vi "read_data (SubVI).vi"(0 "VISA resource name":refnum<visa-resource-name>, 1 "Scope only?":bool=TRUE, 2 "Channels":i32[](array[ring]) items=["Channel 1"=0, "Channel 2"=1, "Channel 3"=2, "Channel 4"=3, "Waveform Memory 1"=5, "Waveform Memory 2"=6, "Serial Bus 1"=7, "Serial Bus 2"=8, "Digital Bus Low"=9, "Digital Bus High "=10, "Digital Bus 1"=11, "Digital Bus 2"=12, "Function 1"=32, "Function 2"=33, "Function 3"=34, "Function 4"=35, "Math 1"=36, "Math 2"=37, "Math 3"=38, "Math 4"=39], 5 "Use osciloscope chan 1":bool, 8 "index (row)":i32, 9 "error in (no error)":errorcluster, 11 "data tasks":T1) -> (4 "output data tasks":T3, 6 "Output data":dbl[][](array[numeric]), 7 "Output ASD 1":cluster{"f0":dbl, "df":dbl, "magnitude":dbl[]}[](array[cluster]), 10 "sample rate":dbl, 12 "Rescaled data":i16[][](array[numeric]), 13 "Output ASD 2":cluster{"f0":dbl, "df":dbl, "magnitude":dbl[]}, 14 "error out":errorcluster, 15 "VISA resource name out":refnum<visa-resource-name>)   [LabVIEW 2018]
uses:
  <vilib>/measure/maspectr.llb/Power Spectrum and PSD Export Mode.ctl
  <vilib>/DAQmx/read.llb/DAQmx Read (Analog 2D DBL NChan NSamp).vi
  <vilib>/DAQmx/miscellaneous.llb/DAQmx Fill In Error Info.vi
  <vilib>/measure/maspectr.llb/FFT Power Spectrum and PSD for 1 Chan.vi
  <vilib>/measure/NI_MAPro.lvlib
panel:
  in  "export mode 3":T2 items=["Power Spectrum", "Power Spectral Density"]
  in  "export mode 2":T2 items=["Power Spectrum", "Power Spectral Density"]
  in  "export mode":T2 items=["Power Spectrum", "Power Spectral Density"]
  out "error out 3":errorcluster
  out "VISA resource name out 3":refnum<visa-resource-name>
  in  "error in (no error) 3":errorcluster
  in  "Channels 3":i32[](array[ring]) items=["Channel 1"=0, "Channel 2"=1, "Channel 3"=2, "Channel 4"=3, "Waveform Memory 1"=5, "Waveform Memory 2"=6, "Serial Bus 1"=7, "Serial Bus 2"=8, "Digital Bus Low"=9, "Digital Bus High "=10, "Digital Bus 1"=11, "Digital Bus 2"=12, "Function 1"=32, "Function 2"=33, "Function 3"=34, "Function 4"=35, "Math 1"=36, "Math 2"=37, "Math 3"=38, "Math 4"=39]
  in  "VISA resource name 3":refnum<visa-resource-name>
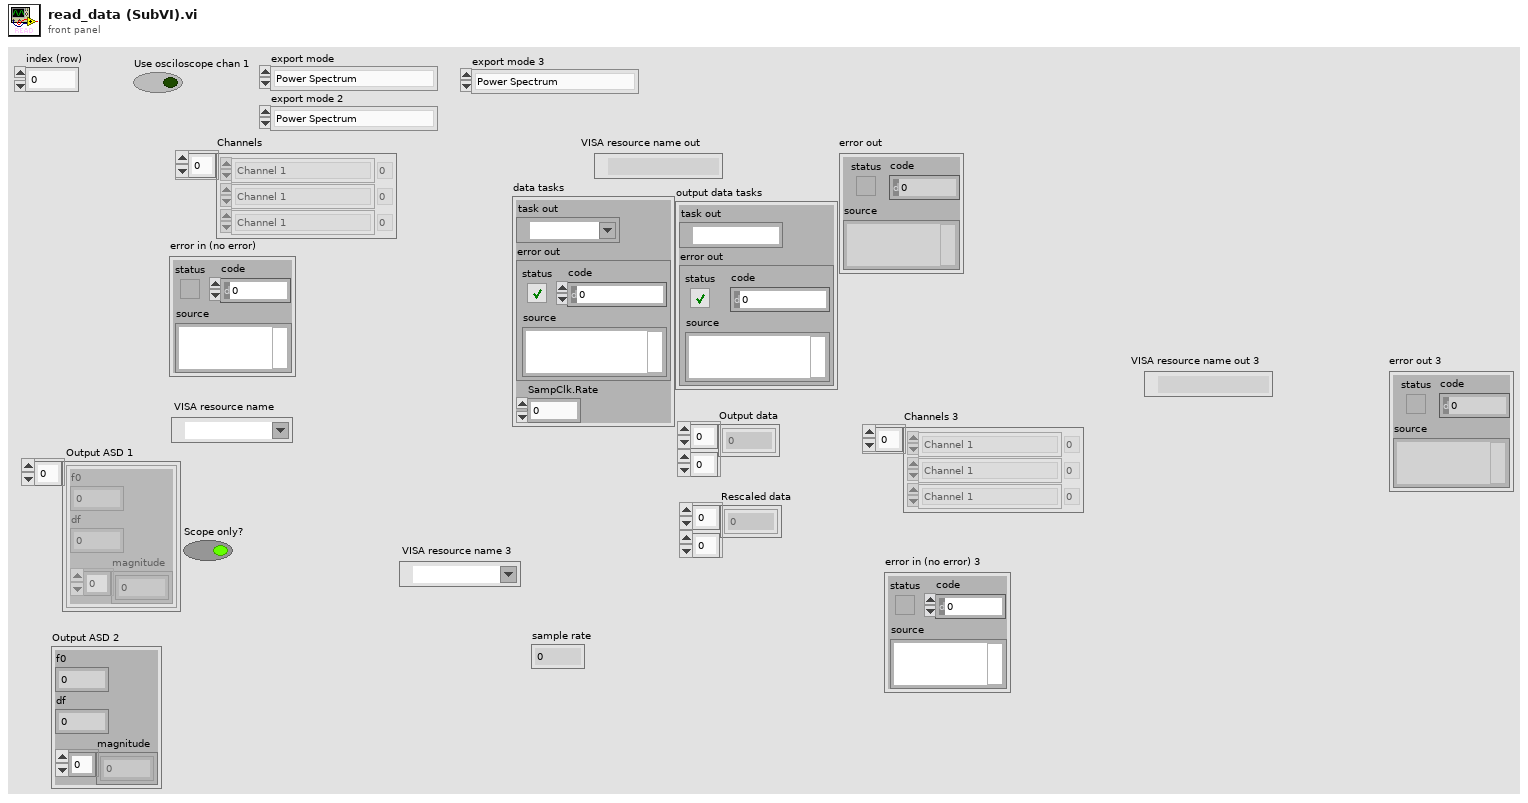
[diagram p1: front panel]
types:
  T1 = cluster{"task out":refnum<k21>, "error out":errorcluster, "SampClk.Rate":dbl}
  T2 = typedef "NI_MAPro.lvlib/Power Spectrum and PSD Export Mode.ctl" = u16
  T3 = cluster{"task out":refnum<k21>, "error out":errorcluster}
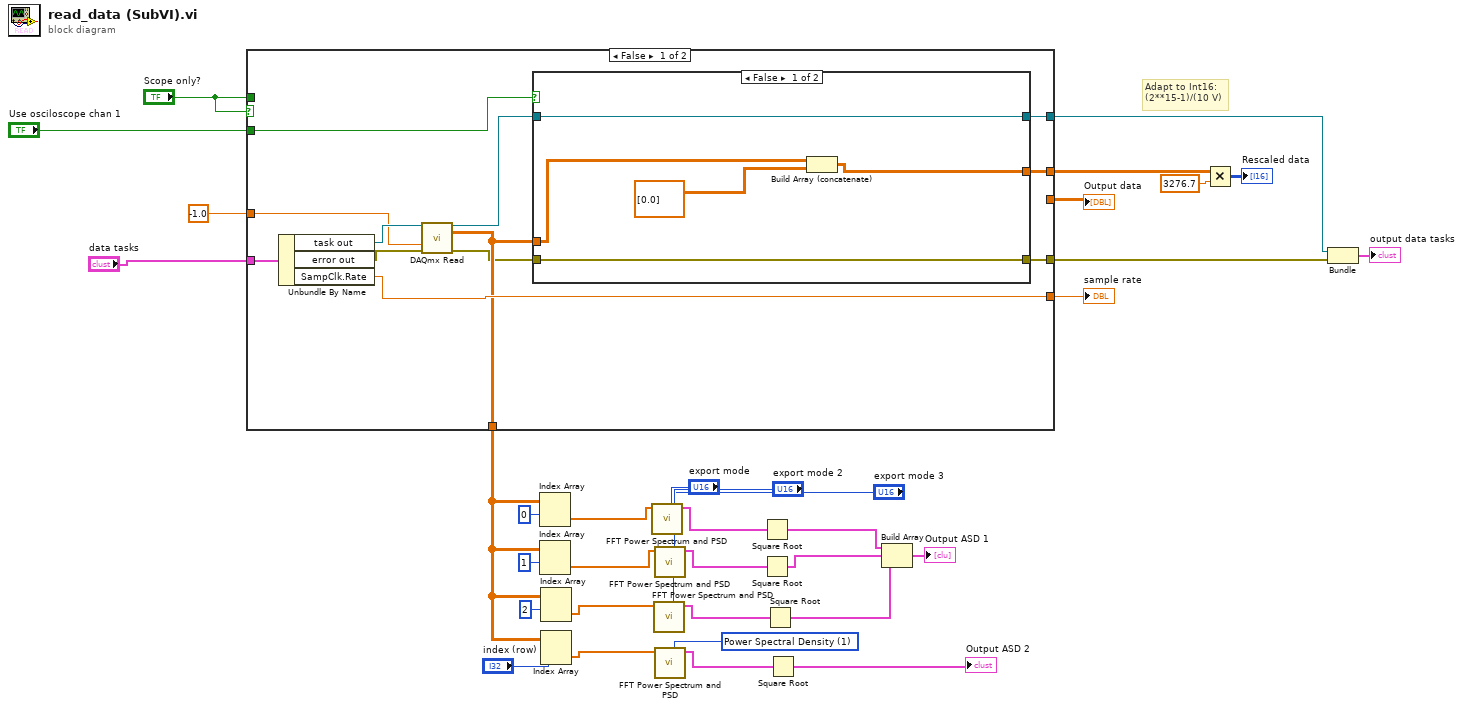
[diagram p0: block diagram]
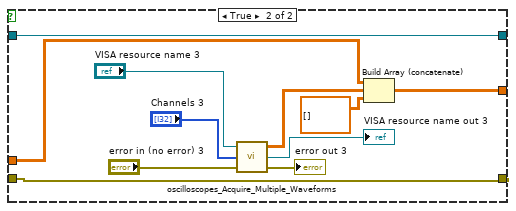
[diagram p2: hidden frame]
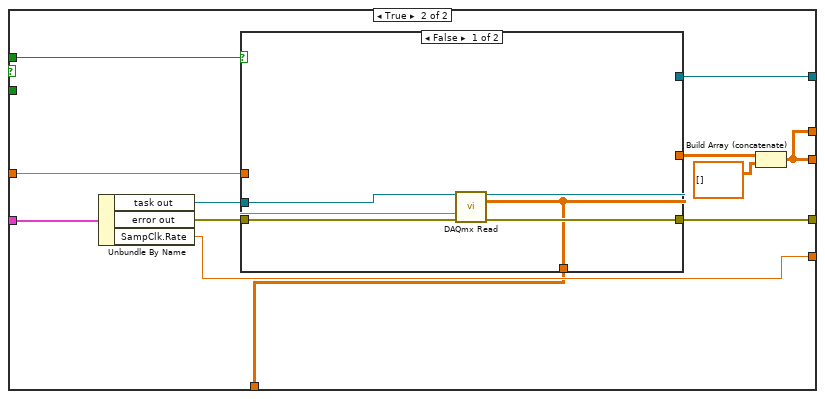
[diagram p3: hidden frame]
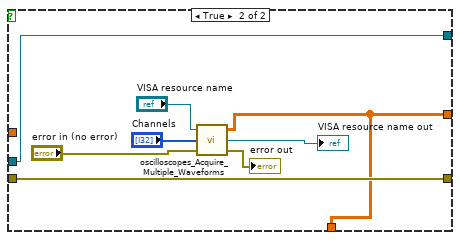
[diagram p4: hidden frame]
diagram:
  w12 = T2 1 items=["Power Spectrum", "Power Spectral Density"] ("export mode")
  # "Adapt to Int16: \n(2**15-1)/(10 V)"
  n1 = case shown="False" "Scope only?" {
    tunnel: "data tasks" -> [w35 w74]
    tunnel: [w40 w70] -> w33
    tunnel: [w39 w69] -> w32
    tunnel: [w41 w65] -> w29
    tunnel: "Use osciloscope chan 1" -> [w42 _]
    tunnel: "Scope only?" -> [_ w67]
    tunnel: [w46 w66] -> w26
    tunnel: [w41 w65] -> w25
    tunnel: -1.0 ("timeout") -> [w43 w64]
    tunnel: [w38 w63] -> w22
    frame False {
      n2 = Unbundle By Name(w35) -> ("task out"=w44:refnum<k21>, "error out"=w45:errorcluster, "SampClk.Rate"=w46:dbl)
      n3 = call-poly <vilib>:"DAQmx Read.vi"("task/channels in"=w44, "timeout"=w43, "error in"=w45) -> ("task out"=w37:refnum<k21>, "data"=w38:dbl[][], "error out"=w36:errorcluster)  [unwired: 10 in]
      n4 = case shown="False" w42 {
        tunnel: w38 -> [w49 w56]
        tunnel: [w48 w55] -> w41
        tunnel: [w51 w53] -> w40
        tunnel: w37 -> [w51 w53]
        tunnel: [w50 w52] -> w39
        tunnel: w36 -> [w50 w52]
        frame False {
          n5 = Build Array (concatenate)(w49, dbl[][] [[0.0]] ("array")) -> (w48:dbl[][])
        }
        frame True {
          n6 = call "oscilloscopes_Acquire_Multiple_Waveforms.vi"("error in (no error)"="error in (no error) 3", "Channels"="Channels 3", "VISA resource name"="VISA resource name 3") -> ("error out"=→"error out 3":errorcluster, "VISA resource name out"=→"VISA resource name out 3":refnum<visa-resource-name>, "Y"=w54:dbl[][])
          n7 = Build Array (concatenate)(w56, w54, dbl[][] [] ("array")) -> (w55:dbl[][])
        }
      }
    }
    frame True {
      n8 = Unbundle By Name(w74) -> ("task out"=w73:refnum<k21>, "error out"=w72:errorcluster, "SampClk.Rate"=w66:dbl)
      n9 = case shown="False" w67 {
        tunnel: w73 -> [w80 w88]
        tunnel: w72 -> [w79 w87]
        tunnel: w64 -> [w78 _]
        tunnel: [w75 w81] -> w71
        tunnel: [w77 w88] -> w70
        tunnel: [w76 w87] -> w69
        tunnel: [w75 w81] -> w63
        frame False {
          n10 = call-poly <vilib>:"DAQmx Read.vi"("task/channels in"=w80, "timeout"=w78, "error in"=w79) -> ("task out"=w77:refnum<k21>, "data"=w75:dbl[][], "error out"=w76:errorcluster)  [unwired: 10 in]
        }
        frame True {
          n11 = call "oscilloscopes_Acquire_Multiple_Waveforms.vi"("error in (no error)"="error in (no error)", "Channels"="Channels", "VISA resource name"="VISA resource name") -> ("error out"=→"error out":errorcluster, "VISA resource name out"=→"VISA resource name out":refnum<visa-resource-name>, "Y"=w81:dbl[][])
        }
      }
      n12 = Build Array (concatenate)(w71, dbl[][] [] ("array")) -> (w65:dbl[][])
    }
  }
  "sample rate" <- w26
  "Output data" <- w25
  n13 = Index Array(array=w22, index (row)=0) -> (element=w18:dbl[])  [unwired: 1 in]
  n14 = Index Array(array=w22, index (row)=1) -> (element=w14:dbl[])  [unwired: 1 in]
  n15 = Index Array(array=w22, index (row)=2) -> (element=w13:dbl[])  [unwired: 1 in]
  n16 = Index Array(array=w22, index (row)="index (row)") -> (element=w11:dbl[])  [unwired: 1 in]
  n17 = call-poly <vilib>:"FFT Power Spectrum and PSD.vi"("export mode"="export mode", "time signal"=w18) -> ("Power Spectrum / PSD"=w9:cluster{"f0":dbl, "df":dbl, "magnitude":dbl[]})  [unwired: 6 in, 3 out]
  n18 = call-poly <vilib>:"FFT Power Spectrum and PSD.vi"("export mode"="export mode 3", "time signal"=w13) -> ("Power Spectrum / PSD"=w7:cluster{"f0":dbl, "df":dbl, "magnitude":dbl[]})  [unwired: 6 in, 3 out]
  n19 = call-poly <vilib>:"FFT Power Spectrum and PSD.vi"("export mode"="export mode 2", "time signal"=w14) -> ("Power Spectrum / PSD"=w8:cluster{"f0":dbl, "df":dbl, "magnitude":dbl[]})  [unwired: 6 in, 3 out]
  n20 = call-poly <vilib>:"FFT Power Spectrum and PSD.vi"("export mode"=w12, "time signal"=w11) -> ("Power Spectrum / PSD"=w3:cluster{"f0":dbl, "df":dbl, "magnitude":dbl[]})  [unwired: 6 in, 3 out]
  n21 = Square Root(x=w9) -> (sqrt(x)=w4:cluster{"f0":dbl, "df":dbl, "magnitude":dbl[]})
  n22 = Square Root(x=w8) -> (sqrt(x)=w5:cluster{"f0":dbl, "df":dbl, "magnitude":dbl[]})
  n23 = Square Root(x=w7) -> (sqrt(x)=w6:cluster{"f0":dbl, "df":dbl, "magnitude":dbl[]})
  n24 = Square Root(x=w3) -> (sqrt(x)=→"Output ASD 2":cluster{"f0":dbl, "df":dbl, "magnitude":dbl[]})
  n25 = Build Array(w4, w5, w6) -> (→"Output ASD 1":cluster{"f0":dbl, "df":dbl, "magnitude":dbl[]}[])
  n26 = Multiply(x=w29, y=3276.7) -> (x*y=→"Rescaled data":i16[][])
  n27 = Bundle("task out"=w33, "error out"=w32) -> (→"output data tasks":T3)  [unwired: 1 in]
